vi "Power Output Plot Measurement.vi"(4 "Measured Values":refnum<vi>, 5 "Minimum Power":cluster{dbl[], dbl[]}, 6 "Reset Plot? (F)":bool, 7 "Plots":T2, 8 "error in (no error)":errorcluster, 9 "Frequency Range (MHz)":cluster{"Start (MHz)":dbl, "Stop (MHz)":dbl}, 11 "Measurement Data":T1) -> (0 "error out":errorcluster)   [LabVIEW 2011]
uses:
  TypeDefs/Power Output Measurement Data.ctl
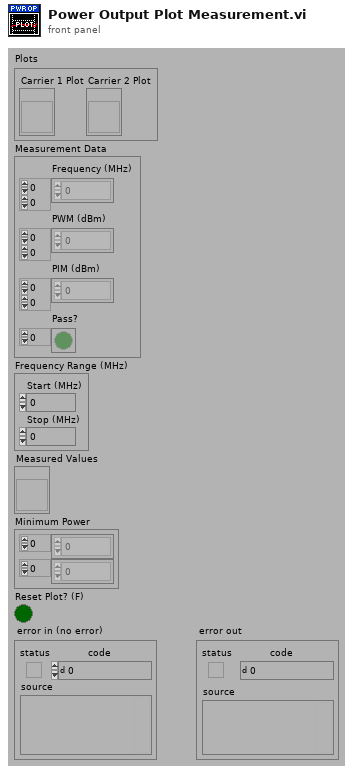
[diagram p1: front panel]
types:
  T1 = typedef "Power Output Measurement Data.ctl" = cluster{"Frequency (MHz)":dbl[][], "PWM (dBm)":dbl[][], "PIM (dBm)":dbl[][], "Pass?":bool[]}
  T2 = cluster{"Carrier 1 Plot":refnum<vi>, "Carrier 2 Plot":refnum<vi>}
  T3 = cluster{"Array Constant":dbl[], "Array Constant":dbl[]}[]
  T4 = cluster{"Frequency (MHz)":dbl[], "PWM (dBm)":dbl[]}
  T5 = cluster{"Frequency (MHz)":dbl[], "PIM (dBm)":dbl[]}
  T6 = cluster{"Frequency (MHz)":dbl[], "PIM (dBm)":dbl[]}[]
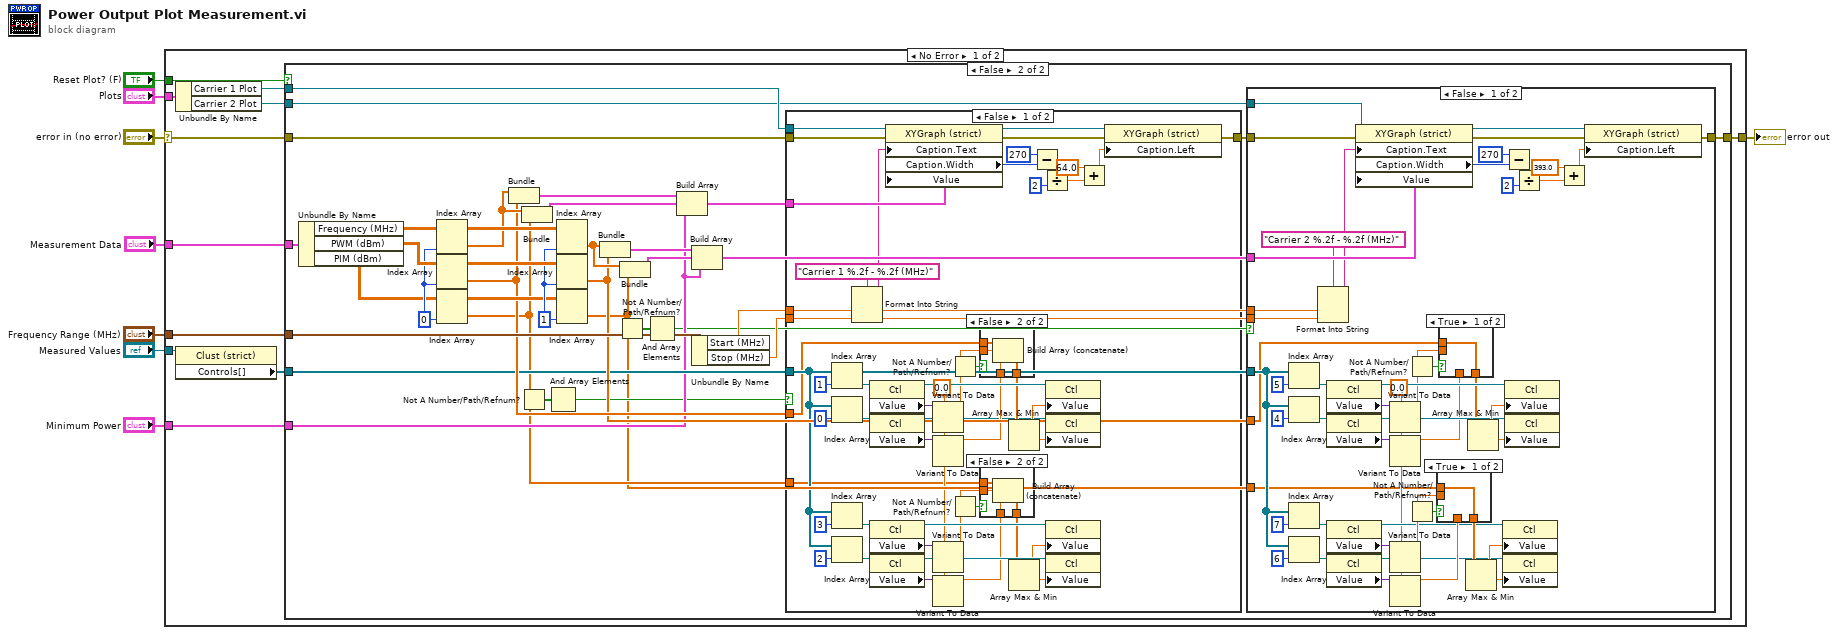
[diagram p0: block diagram]
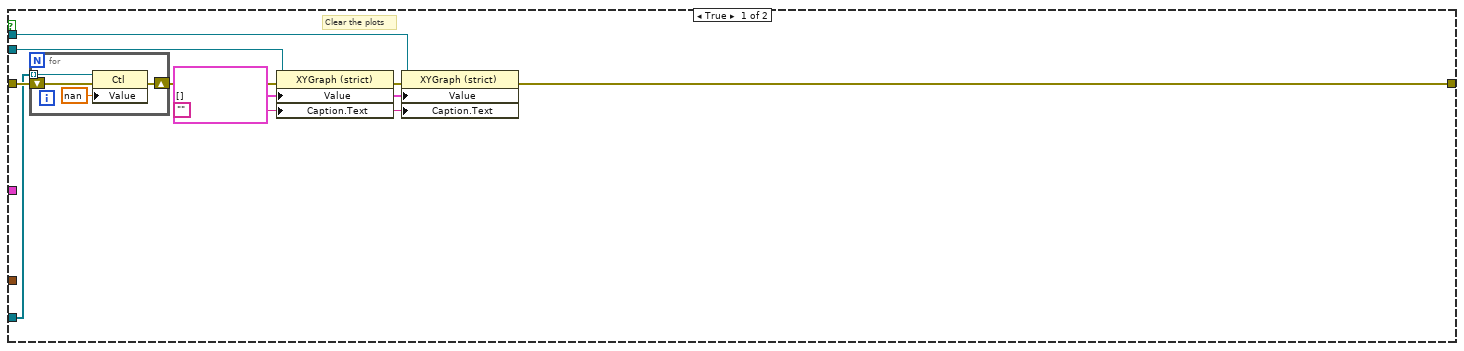
[diagram p2: hidden frame]
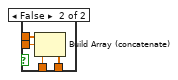
[diagram p3: hidden frame]
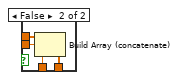
[diagram p4: hidden frame]
diagram:
  n1 = case shown="No Error" "error in (no error)" {
    selector: "error in (no error)" -> [w19 w184]
    tunnel: "Reset Plot? (F)" -> [w11 _]
    tunnel: [w14 w184] -> w7
    tunnel: "Measurement Data" -> [w18 _]
    tunnel: "Minimum Power" -> [w13 _]
    tunnel: "Plots" -> [w17 _]
    tunnel: "Measured Values" -> [w10 _]
    tunnel: "Frequency Range (MHz)" -> [w12 _]
    frame No Error {
      n2 = Unbundle By Name(w17) -> ("Carrier 1 Plot"=w16:refnum<vi>, "Carrier 2 Plot"=w15:refnum<vi>)
      n3 = property class="Clust (strict)"(reference=w10) -> ("Controls[]"=w9:refnum<vi>[])  [unwired: 1 in, 2 out]
      n4 = case shown="False" w11 {
        tunnel: w19 -> [w28 w41]
        tunnel: w18 -> [_ w63]
        tunnel: w16 -> [w27 w42]
        tunnel: w15 -> [w26 w40]
        tunnel: [w25 w62] -> w14
        tunnel: w13 -> [_ w39]
        tunnel: w12 -> [_ w61]
        tunnel: w9 -> [w24 w43]
        frame True {
          w20 = ""
          w22 = T3 [] ("Value")
          # "Clear the plots"
          n5 = for {
            shift-right: [w31] -> w21
            shift-left: w28 -> [w32]
            tunnel: w24 -> [w30] mode=indexing
            n6 = property class="Ctl"(reference=w30, error in=w32, "Value"=nan) -> (error out=w31:errorcluster)  [unwired: 1 out]
          }
          n7 = property class="XYGraph (strict)"(reference=w26, error in=w21, "Value"=w22, "Caption.Text"=w20) -> (error out=w23:errorcluster)  [unwired: 1 out]
          n8 = property class="XYGraph (strict)"(reference=w27, error in=w23, "Value"=w22, "Caption.Text"=w20) -> (error out=w25:errorcluster)  [unwired: 1 out]
        }
        frame False {
          w53 = 1 ("disabled index (col)")
          w54 = 0 ("disabled index (col)")
          n9 = Unbundle By Name(w63) -> ("Frequency (MHz)"=w57:dbl[][], "PWM (dBm)"=w56:dbl[][], "PIM (dBm)"=w52:dbl[][])
          n10 = Index Array(array=w57, index (col)=w54) -> (element=w49:dbl[])  [unwired: 1 in]
          n11 = Index Array(array=w56, index (col)=w54) -> (element=w45:dbl[])  [unwired: 1 in]
          n12 = Index Array(array=w52, index (col)=w54) -> (element=w38:dbl[])  [unwired: 1 in]
          n13 = Bundle("Frequency (MHz)"=w49, "PWM (dBm)"=w45) -> (w59:T4)  [unwired: 1 in]
          n14 = Not A Number/Path/Refnum?(number/path/refnum=w38) -> (NaN/Path/Refnum?=w37:bool[])
          n15 = Bundle("Frequency (MHz)"=w49, "PIM (dBm)"=w38) -> (w55:T5)  [unwired: 1 in]
          n16 = And Array Elements(Boolean array=w37) -> (logical AND=w36:bool)
          n17 = Index Array(array=w57, index (col)=w53) -> (element=w48:dbl[])  [unwired: 1 in]
          n18 = Index Array(array=w56, index (col)=w53) -> (element=w44:dbl[])  [unwired: 1 in]
          n19 = Index Array(array=w52, index (col)=w53) -> (element=w35:dbl[])  [unwired: 1 in]
          n20 = Bundle("Frequency (MHz)"=w48, "PWM (dBm)"=w44) -> (w50:T4)  [unwired: 1 in]
          n21 = Not A Number/Path/Refnum?(number/path/refnum=w35) -> (NaN/Path/Refnum?=w34:bool[])
          n22 = Bundle("Frequency (MHz)"=w48, "PIM (dBm)"=w35) -> (w51:T5)  [unwired: 1 in]
          n23 = And Array Elements(Boolean array=w34) -> (logical AND=w33:bool)
          n24 = Build Array(w59, w55, w39) -> (w60:T6)
          n25 = Build Array(w50, w51, w39) -> (w58:T6)
          n26 = Unbundle By Name(w61) -> ("Start (MHz)"=w47:dbl, "Stop (MHz)"=w46:dbl)
          n27 = case shown="False" w36 {
            tunnel: w42 -> [w172 _]
            tunnel: [w126 w183] -> w62
            tunnel: w41 -> [w171 w183]
            tunnel: w60 -> [w170 _]
            tunnel: w43 -> [w140 _]
            tunnel: w47 -> [w153 _]
            tunnel: w46 -> [w152 _]
            tunnel: w45 -> [w151 _]
            tunnel: w38 -> [w134 _]
            frame False {
              w139 = 0.0
              n28 = Index Array(array=w140, index=1) -> (element=w167:refnum<vi>)
              n29 = Index Array(array=w140, index=0) -> (element=w166:refnum<vi>)
              n30 = Index Array(array=w140, index=3) -> (element=w143:refnum<vi>)
              n31 = Index Array(array=w140, index=2) -> (element=w144:refnum<vi>)
              n32 = Format Into String(format string="Carrier 1 %.2f - %.2f (MHz)", w153, w152) -> (resulting string=w154:string)  [unwired: 2 in, 1 out]
              n33 = property class="Ctl"(reference=w167) -> (reference out=w165:refnum<vi>, "Value"=w164:variant)  [unwired: 1 in, 1 out]
              n34 = property class="Ctl"(reference=w166) -> (reference out=w159:refnum<vi>, "Value"=w163:variant)  [unwired: 1 in, 1 out]
              n35 = property class="Ctl"(reference=w143) -> (reference out=w145:refnum<vi>, "Value"=w146:variant)  [unwired: 1 in, 1 out]
              n36 = property class="Ctl"(reference=w144) -> (reference out=w149:refnum<vi>, "Value"=w147:variant)  [unwired: 1 in, 1 out]
              n37 = property class="XYGraph (strict)"(reference=w172, error in=w171, "Caption.Text"=w154, "Value"=w170) -> (reference out=w125:refnum<vi>, error out=w127:errorcluster, "Caption.Width"=w133:u32)
              n38 = Variant To Data(type=w139, Variant=w164) -> (data=w156:dbl)  [unwired: 1 in, 1 out]
              n39 = Variant To Data(type=w139, Variant=w163) -> (data=w162:dbl)  [unwired: 1 in, 1 out]
              n40 = Variant To Data(type=w139, Variant=w146) -> (data=w137:dbl)  [unwired: 1 in, 1 out]
              n41 = Variant To Data(type=w139, Variant=w147) -> (data=w136:dbl)  [unwired: 1 in, 1 out]
              n42 = Not A Number/Path/Refnum?(number/path/refnum=w156) -> (NaN/Path/Refnum?=w157:bool)
              n43 = Not A Number/Path/Refnum?(number/path/refnum=w137) -> (NaN/Path/Refnum?=w138:bool)
              n44 = case shown="False" w157 {
                tunnel: w162 -> [_ w182]
                tunnel: [w178 w181] -> w161
                tunnel: w151 -> [w178 w180]
                tunnel: w156 -> [_ w179]
                frame True {
                }
                frame False {
                  n45 = Build Array (concatenate)(w180, w179, w182) -> (w181:dbl[])
                }
              }
              n46 = case shown="False" w138 {
                tunnel: w136 -> [_ w177]
                tunnel: [w173 w176] -> w135
                tunnel: w134 -> [w173 w175]
                tunnel: w137 -> [_ w174]
                frame True {
                }
                frame False {
                  n47 = Build Array (concatenate)(w175, w174, w177) -> (w176:dbl[])
                }
              }
              n48 = Array Max & Min(array=w161) -> (max value=w160:dbl, min value=w158:dbl)  [unwired: 2 out]
              n49 = Array Max & Min(array=w135) -> (max value=w148:dbl, min value=w150:dbl)  [unwired: 2 out]
              n50 = Subtract(x=u32 270, y=w133) -> (x-y=w131:u32)
              n51 = Divide(x=w131, y=u32 2) -> (x/y=w129:dbl)
              n52 = property class="Ctl"(reference=w165, "Value"=w160) -> ()  [unwired: 1 in, 2 out]
              n53 = property class="Ctl"(reference=w159, "Value"=w158) -> ()  [unwired: 1 in, 2 out]
              n54 = property class="Ctl"(reference=w145, "Value"=w148) -> ()  [unwired: 1 in, 2 out]
              n55 = property class="Ctl"(reference=w149, "Value"=w150) -> ()  [unwired: 1 in, 2 out]
              n56 = Add(x=64.0, y=w129) -> (x+y=w124:dbl)
              n57 = property class="XYGraph (strict)"(reference=w125, error in=w127, "Caption.Left"=w124) -> (error out=w126:errorcluster)  [unwired: 1 out]
            }
            frame True {
            }
          }
          n58 = case shown="False" w33 {
            tunnel: [w66 w123] -> _
            tunnel: w62 -> [w112 w123]
            tunnel: w58 -> [w111 _]
            tunnel: w43 -> [w76 _]
            tunnel: w40 -> [w100 _]
            tunnel: w47 -> [w94 _]
            tunnel: w46 -> [w92 _]
            tunnel: w44 -> [w75 _]
            tunnel: w35 -> [w74 _]
            frame False {
              w77 = 0.0
              n59 = Index Array(array=w76, index=5) -> (element=w108:refnum<vi>)
              n60 = Index Array(array=w76, index=4) -> (element=w107:refnum<vi>)
              n61 = Index Array(array=w76, index=7) -> (element=w85:refnum<vi>)
              n62 = Index Array(array=w76, index=6) -> (element=w84:refnum<vi>)
              n63 = Format Into String(format string="Carrier 2 %.2f - %.2f (MHz)", w94, w92) -> (resulting string=w93:string)  [unwired: 2 in, 1 out]
              n64 = property class="Ctl"(reference=w108) -> (reference out=w106:refnum<vi>, "Value"=w105:variant)  [unwired: 1 in, 1 out]
              n65 = property class="Ctl"(reference=w107) -> (reference out=w102:refnum<vi>, "Value"=w104:variant)  [unwired: 1 in, 1 out]
              n66 = property class="Ctl"(reference=w85) -> (reference out=w83:refnum<vi>, "Value"=w82:variant)  [unwired: 1 in, 1 out]
              n67 = property class="Ctl"(reference=w84) -> (reference out=w79:refnum<vi>, "Value"=w81:variant)  [unwired: 1 in, 1 out]
              n68 = property class="XYGraph (strict)"(reference=w100, error in=w112, "Caption.Text"=w93, "Value"=w111) -> (reference out=w65:refnum<vi>, error out=w67:errorcluster, "Caption.Width"=w64:u32)
              n69 = Variant To Data(type=w77, Variant=w105) -> (data=w96:dbl)  [unwired: 1 in, 1 out]
              n70 = Variant To Data(type=w77, Variant=w104) -> (data=w98:dbl)  [unwired: 1 in, 1 out]
              n71 = Variant To Data(type=w77, Variant=w82) -> (data=w89:dbl)  [unwired: 1 in, 1 out]
              n72 = Variant To Data(type=w77, Variant=w81) -> (data=w90:dbl)  [unwired: 1 in, 1 out]
              n73 = Not A Number/Path/Refnum?(number/path/refnum=w96) -> (NaN/Path/Refnum?=w97:bool)
              n74 = Not A Number/Path/Refnum?(number/path/refnum=w89) -> (NaN/Path/Refnum?=w88:bool)
              n75 = case shown="True" w88 {
                tunnel: w90 -> [_ w117]
                tunnel: [w113 w116] -> w91
                tunnel: w74 -> [w113 w115]
                tunnel: w89 -> [_ w114]
                frame True {
                }
                frame False {
                  n76 = Build Array (concatenate)(w115, w114, w117) -> (w116:dbl[])
                }
              }
              n77 = case shown="True" w97 {
                tunnel: w98 -> [_ w122]
                tunnel: [w118 w121] -> w99
                tunnel: w75 -> [w118 w120]
                tunnel: w96 -> [_ w119]
                frame True {
                }
                frame False {
                  n78 = Build Array (concatenate)(w120, w119, w122) -> (w121:dbl[])
                }
              }
              n79 = Array Max & Min(array=w91) -> (max value=w80:dbl, min value=w78:dbl)  [unwired: 2 out]
              n80 = Array Max & Min(array=w99) -> (max value=w103:dbl, min value=w101:dbl)  [unwired: 2 out]
              n81 = property class="Ctl"(reference=w83, "Value"=w80) -> ()  [unwired: 1 in, 2 out]
              n82 = property class="Ctl"(reference=w79, "Value"=w78) -> ()  [unwired: 1 in, 2 out]
              n83 = Subtract(x=u32 270, y=w64) -> (x-y=w69:u32)
              n84 = property class="Ctl"(reference=w106, "Value"=w103) -> ()  [unwired: 1 in, 2 out]
              n85 = property class="Ctl"(reference=w102, "Value"=w101) -> ()  [unwired: 1 in, 2 out]
              n86 = Divide(x=w69, y=u32 2) -> (x/y=w71:dbl)
              n87 = Add(x=393.0, y=w71) -> (x+y=w73:dbl)
              n88 = property class="XYGraph (strict)"(reference=w65, error in=w67, "Caption.Left"=w73) -> (error out=w66:errorcluster)  [unwired: 1 out]
            }
            frame True {
            }
          }
        }
      }
    }
    frame Error {
    }
  }
  "error out" <- w7
